vi "Format Error.vi"(3 "input cluster":errorcluster) -> (1 "resulting string":string)   [LabVIEW 2019, in "Sports Unit Tests.lvclass"]
uses:
  Sports Unit Tests.lvclass
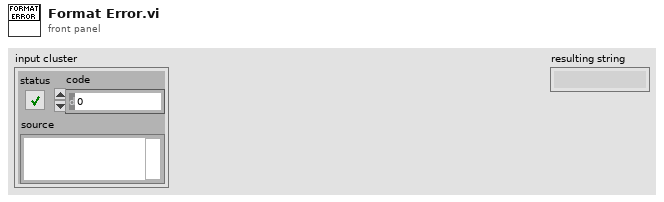
[diagram p1: front panel]
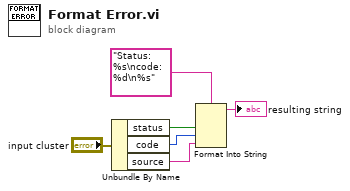
[diagram p0: block diagram]
diagram:
  n1 = Unbundle By Name("input cluster") -> ("status"=w6:bool, "code"=w5:i32, "source"=w4:string)
  n2 = Format Into String(format string="Status: %s\ncode: %d\n%s", w6, w5, w4) -> (resulting string=→"resulting string":string)  [unwired: 2 in, 1 out]
